vi "String Split at Count.vi"(2 "# of characters in 1st string":i32, 3 "String to Split":string) -> (0 "2nd String":string, 1 "1st String":string)   [LabVIEW 2016, in "eec EST 300.lvlib"]
uses:
  <instrlib>/eec EST 300/eec EST 300.lvlib
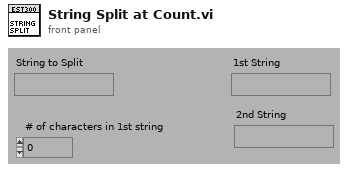
[diagram p1: front panel]
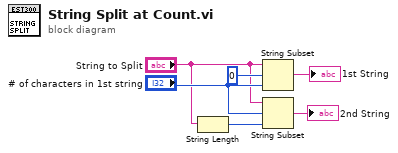
[diagram p0: block diagram]
diagram:
  n1 = String Length(string="String to Split") -> (length=w3:i32)
  n2 = String Subset ("截取字符串")(string="String to Split", offset (0)=0, length (rest)="# of characters in 1st string") -> (substring=→"1st String":string)
  n3 = String Subset(string="String to Split", offset (0)="# of characters in 1st string", length (rest)=w3) -> (substring=→"2nd String":string)
